vi "GetPixelToGantryCoordinates.vi"(3 "error in (no error)":errorcluster, 4 "PixelY":dbl, 5 "PixelX":dbl) -> (0 "error out":errorcluster, 1 "YmmGH":dbl, 2 "XmmGH":dbl)   [LabVIEW 2019]
panel:
  out "Coord":dbl
  out "Program Position U":dbl
  out "Position U":dbl
  out "Velocity U":dbl
  out "Program Position Z":dbl
  out "Position Z":dbl
  out "Velocity Z":dbl
  out "Program Position Y":dbl
  out "Position Y":dbl
  out "Velocity Y":dbl
  out "Program Position X":dbl
  out "Position X":dbl
  out "Velocity X":dbl format="%#.5g"
  in  "GHtoCamOffsetYmm":dbl=117.045
  in  "GHtoCamOffsetXmm":dbl=29.795
  out "XmmRelGH":dbl
  out "YmmRelGH":dbl
  in  "NPixelsY":dbl=1920.0
  in  "NPixelsX":dbl=2560.0
  in  "MicronsPerPixel":dbl=0.4348
  # "Convert pixels to X and Y relative to gantry head (GH). Units of X & Y are in mm."
  # "Constants here"
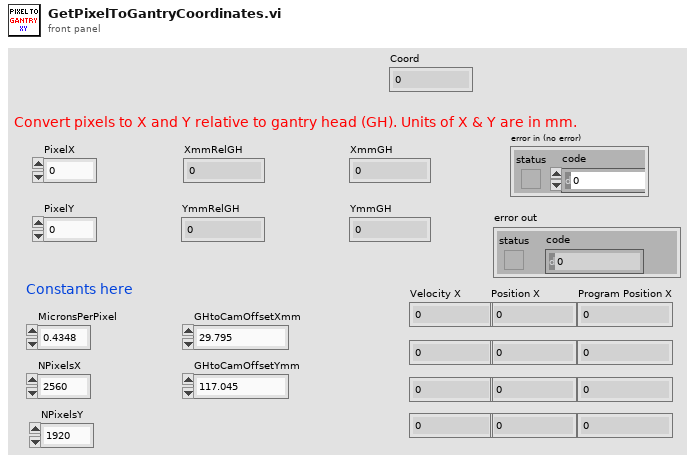
[diagram p1: front panel]
types:
  T1 = typedef "ControllerDiagPacket.ctl" = cluster{"Number of Diag Packets":i32, "Axes":T2[], "error":errorcluster}
  T2 = typedef "AxisDiagPacket.ctl" = cluster{"Axis Name":string, "Analog Input 0":dbl, "Analog Input 1":dbl, "Axis Fault (num)":i32, "Axis Fault (str)":string, "Axis Fault (bits)":cluster{"AmplifierFault":bool, "AmplifierTemperatureFault":bool, "CcwEndOfTravelLimitFault":bool, "CcwSoftwareLimitFault":bool, "CommunicationLostFault":bool, "CwEndOfTravelLimitFault":bool, "CwSoftwareLimitFault":bool, "EmergencyStopFault":bool, "EncoderFault":bool, "ExternalFault":bool, "FeedbackScalingFault":bool, "GantryMisalignFault ":bool, "HallSensorFault":bool, "InPositionTimeoutFault":bool, "InternalFault":bool, "MarkerSearchFault":bool, "MaxVelocityCommandFault":bool, "MissedInterruptFault":bool, "MotorTemperatureFault":bool, "None":bool, "OverCurrentFault":bool, "PositionErrorFault":bool, "PositionFeedbackFault":bool, "PowerSupplyFault":bool, "ProbeInputFault":bool, "SafeZoneFault":bool, "VelocityErrorFault":bool, "VelocityFeedbackFault":bool, "VoltageClampFault":bool}, "Axis Status (num)":i32, "Axis Status (str)":string, "Axis Status (bits)":cluster{"BacklashActive":bool, "CalibrationEnabled1D":bool, "CalibrationEnabled2D":bool, "CommandValid":bool, "DriveAbortPending":bool, "DrivePending":bool, "Enabling":bool, "GainMappingEnabled":bool, "GantryAligned":bool, "GantryRealigning":bool, "Homed":bool, "Homing":bool, "IFOVEnabled":bool, "JogGenerating":bool, "Jogging":bool, "JoystickControl":bool, "MasterSlaveControl":bool, "MotionBlocked":bool, "MotionClamped":bool, "MoveDone":bool, "None":bool, "NotVirtual":bool, "Profiling":bool, "Stability0":bool, "Stability1":bool, "TrajectoryFiltering":bool, "WaitDone":bool}, "Current Command":sgl, "Current Error":sgl, "Current Feedback":sgl, "Digital Inputs":i32, "Digital Outputs":i32, "Drive Status":i32, "Drive Status (str)":string, "Drive Status (bits)":cluster{"AccelerationPhase":bool, "AutofocusActive":bool, "BrakeOutput":bool, "CcwEndOfTravelLimitInput":bool, "CosineEncoderError":bool, "CurrentClamp":bool, "CwEndOfTravelLimitInput":bool, "DecelerationPhase":bool, "DualLoopActive":bool, "EmergencyStopInput":bool, "Enabled":bool, "EncoderClipping":bool, "GalvoCalibrationEnabled":bool, "GalvoPowerCorrection":bool, "HallAInput":bool, "HallBInput":bool, "HallCInput":bool, "HighResolutionMode":bool, "HomeLimitInput":bool, "InPosition":bool, "InPosition2":bool, "MarkerInput":bool, "MarkerLatch":bool, "MoveActive":bool, "NoMotorSupply":bool, "None":bool, "PowerLimiting":bool, "ProgrammingFlash":bool, "ProgrammingMXH":bool, "PSOHaltLatch":bool, "ServoControl":bool, "SineEncoderError":bool}, "Position Feedback Auxiliary":dbl, "Position Command":dbl, "Position Error":dbl, "Position Feedback":dbl, "Program Position Command":dbl, "Program Position Error":dbl, "Program Position Feedback":dbl, "Velocity Command":dbl, "Velocity Error":dbl, "Velocity Feedback":dbl}
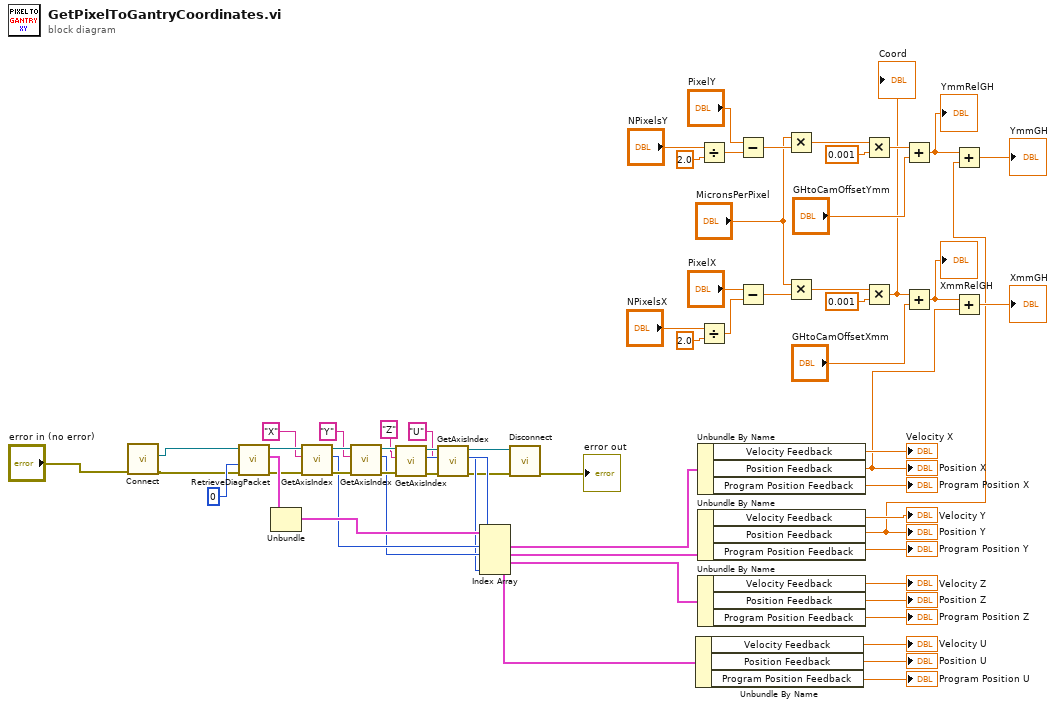
[diagram p0: block diagram]
diagram:
  n1 = call "Connect.vi"("error in (no error)"="error in (no error)") -> ("error out"=w15:errorcluster, "controller"=w14:refnum<k24>)  [unwired: 9 in]
  n2 = call "RetrieveDiagPacket.vi"("error in (no error)"=w15, "axisMask"=0, "Controller In"=w14) -> ("error out"=w46:errorcluster, "ControllerDiagPacket"=w47:T1, "Controller Out"=w45:refnum<k24>)  [unwired: 6 in]
  n3 = Unbundle(w47) -> ("Axes"=w38:T2[])  [unwired: 2 out]
  n4 = call "GetAxisIndex.vi"("error in (no error)"=w46, "axis name"="X", "controller in"=w45) -> ("error out"=w42:errorcluster, "axis index"=w37:i32, "controller out"=w44:refnum<k24>)  [unwired: 6 in]
  n5 = call "GetAxisIndex.vi"("error in (no error)"=w42, "axis name"="Y", "controller in"=w44) -> ("error out"=w41:errorcluster, "axis index"=w36:i32, "controller out"=w43:refnum<k24>)  [unwired: 6 in]
  n6 = call "GetAxisIndex.vi"("error in (no error)"=w41, "axis name"="Z", "controller in"=w43) -> ("error out"=w13:errorcluster, "axis index"=w35:i32, "controller out"=w22:refnum<k24>)  [unwired: 6 in]
  n7 = call "GetAxisIndex.vi"("error in (no error)"=w13, "axis name"="U", "controller in"=w22) -> ("error out"=w11:errorcluster, "axis index"=w20:i32, "controller out"=w12:refnum<k24>)  [unwired: 6 in]
  n8 = Index Array(array=w38, index #1=w37, index #2=w36, index #3=w35, index #4=w20) -> (element #1=w33:T2, element #2=w31:T2, element #3=w32:T2, element #4=w19:T2)
  n9 = call "Disconnect.vi"("error in (no error)"=w11, "controller"=w12) -> ("error out"=→"error out":errorcluster)  [unwired: 9 in]
  n10 = Unbundle By Name(w19) -> ("Velocity Feedback"=→"Velocity U":dbl, "Position Feedback"=→"Position U":dbl, "Program Position Feedback"=→"Program Position U":dbl)
  n11 = Unbundle By Name(w33) -> ("Velocity Feedback"=→"Velocity X":dbl, "Position Feedback"=w6:dbl, "Program Position Feedback"=→"Program Position X":dbl)
  "Position X" <- w6
  n12 = Unbundle By Name(w31) -> ("Velocity Feedback"=→"Velocity Y":dbl, "Position Feedback"=w5:dbl, "Program Position Feedback"=→"Program Position Y":dbl)
  "Position Y" <- w5
  n13 = Unbundle By Name(w32) -> ("Velocity Feedback"=→"Velocity Z":dbl, "Position Feedback"=→"Position Z":dbl, "Program Position Feedback"=→"Program Position Z":dbl)
  n14 = Divide(x="NPixelsY", y=2.0) -> (x/y=w57:dbl)
  n15 = Divide(x="NPixelsX", y=2.0) -> (x/y=w59:dbl)
  n16 = Subtract(x="PixelY", y=w57) -> (x-y=w55:dbl)
  n17 = Subtract(x="PixelX", y=w59) -> (x-y=w56:dbl)
  n18 = Multiply(x="MicronsPerPixel", y=w55) -> (x*y=w48:dbl)
  n19 = Multiply(x="MicronsPerPixel", y=w56) -> (x*y=w50:dbl)
  n20 = Multiply(x=w48, y=0.001) -> (x*y=w4:dbl)
  n21 = Multiply(x=w50, y=0.001) -> (x*y=w3:dbl)
  "Coord" <- w3
  n22 = Add(x=w4, y="GHtoCamOffsetYmm") -> (x+y=w9:dbl)
  "YmmRelGH" <- w9
  n23 = Add(x=w3, y="GHtoCamOffsetXmm") -> (x+y=w10:dbl)
  "XmmRelGH" <- w10
  n24 = Add(x=w9, y=w5) -> (x+y=→"YmmGH":dbl)
  n25 = Add(x=w10, y=w6) -> (x+y=→"XmmGH":dbl)
